vi "Scrap_code-Do_not_use.vi"() -> ()   [LabVIEW 2020]
panel:
  out "transposed array":dbl[][](array[numeric])
  out "OscVoltage":dbl
  in  "error in (no error)":errorcluster
  in  "Min Voltage":dbl
  in  "Max Voltage":dbl
  out "error IO":errorcluster
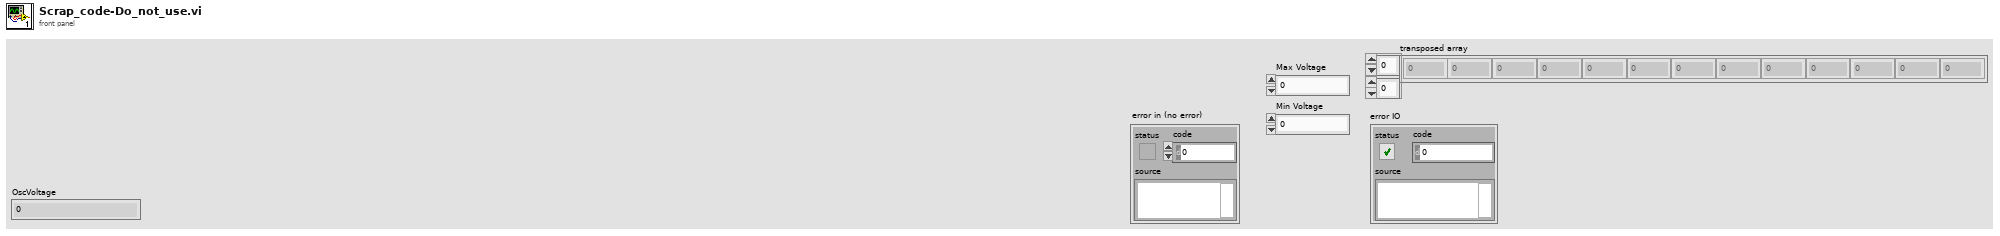
[diagram p1: front panel]
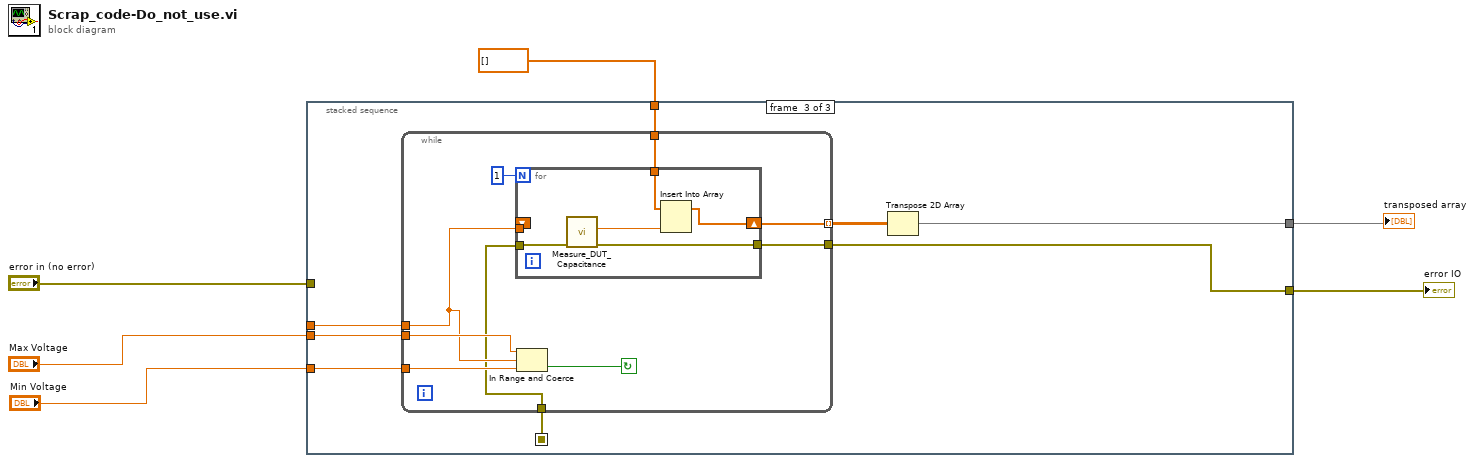
[diagram p0: block diagram]
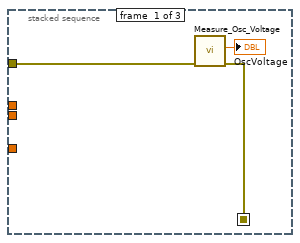
[diagram p2: hidden frame]
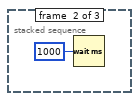
[diagram p3: hidden frame]
diagram:
  n1 = stacked-sequence {
    seq-local: [w7 _ _] -> [_ _ w17]
    tunnel: "error in (no error)" -> [w8 _ _]
    tunnel: _ -> [_ _ w18]
    tunnel: "Max Voltage" -> [_ _ w16]
    tunnel: "Min Voltage" -> [_ _ w15]
    tunnel: dbl[] [] ("array") -> [_ _ w13]
    tunnel: [_ _ w12] -> w2
    tunnel: [_ _ w11] -> w1
    frame #0 {
      n2 = call "Measure_Osc_Voltage.vi"("error in"=w8) -> ("error out"=w7:errorcluster, "OscVoltage"=→"OscVoltage":dbl)  [unwired: 9 in]
    }
    frame #1 {
      n3 = Wait (ms)(milliseconds to wait=u32 1000) -> ()  [unwired: 1 out]
    }
    frame #2 {
      n4 = while {
        tunnel: w18 -> [w23]
        tunnel: w17 -> [w22]
        tunnel: [w20] -> w14 mode=indexing
        tunnel: w16 -> [w25]
        tunnel: w15 -> [w24]
        tunnel: [w21] -> w11
        tunnel: w13 -> [w19]
        stop <- w26 continue-if-true
        n5 = for {
          N: 1 -> [_]
          tunnel: w23 -> [_]
          tunnel: w22 -> [w30]
          tunnel: [w29] -> w21
          shift-right: [w32] -> w20
          shift-left: _ -> [_]
          tunnel: w19 -> [w31]
          n6 = call "Measure_DUT_Capacitance.vi"("error in"=w30) -> ("error out"=w29:errorcluster, "Capacitance Data (in pF)"=w28:dbl)  [unwired: 9 in]
          n7 = Insert Into Array(array=w31, new element=w28) -> (w32:dbl[])  [unwired: 1 in]
        }
        n8 = In Range and Coerce(upper limit=w25, x=w23, lower limit=w24) -> (In Range?=w26:bool)  [unwired: 1 out]
      }
      n9 = Transpose 2D Array(2D array=w14) -> (transposed array=w12:dbl[][])
    }
  }
  "error IO" <- w1
  "transposed array" <- w2
